vi "DisposeCore.vi"(8 "error in (no error)":errorcluster, 11 "PizzaStore":refnum<class "PizzaStore.lvclass">) -> (0 "error out":errorcluster, 3 "PizzaStore":refnum<class "PizzaStore.lvclass">)   [LabVIEW 2020, in "FactoryMethod.lvlib" / "PizzaFactoryMethod.lvlib" / "PizzaStore.lvclass"]
uses:
  PizzaStore.lvclass
  PizzaStore.lvclass/PizzaStore.ctl
  Private/TypeDef/privateDataDVR.ctl
  Private/TypeDef/privateData.ctl
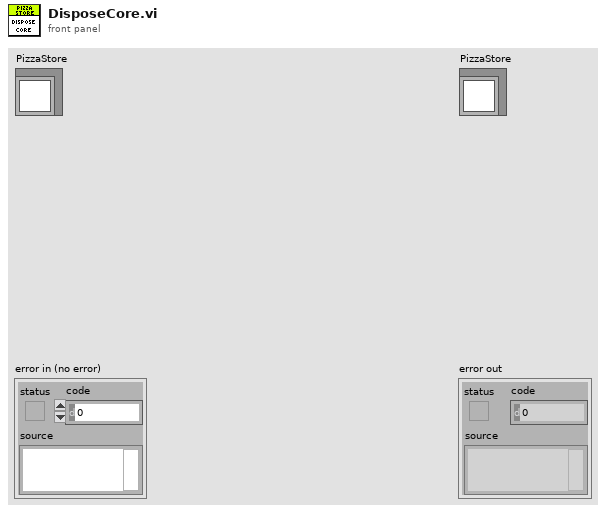
[diagram p1: front panel]
types:
  T1 = typedef "FactoryMethod.lvlib/PizzaFactoryMethod.lvlib/PizzaStore.lvclass/privateDataDVR.ctl" = refnum<data-value>
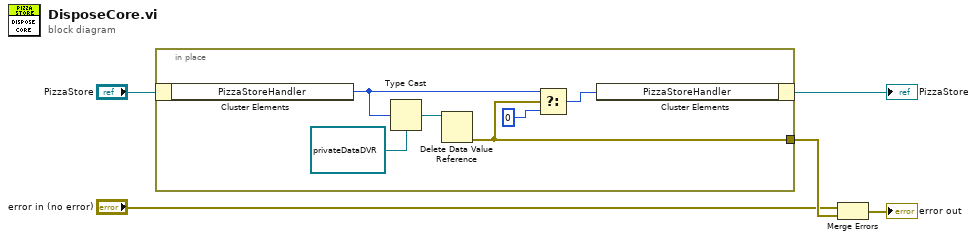
[diagram p0: block diagram]
diagram:
  n1 = in-place {
    in-place-border: [w10] -> w2
    n2 = in-place-cluster #1("PizzaStore") -> ("PizzaStoreHandler"=w9:u32)
    n3 = Type Cast(type=T1 refnum ("privateDataDVR"), x=w9) -> (*(type *) &x=w11:T1)
    n4 = Delete Data Value Reference(data value reference=w11) -> (error out=w10:errorcluster)  [unwired: 1 in, 1 out]
    n5 = Select(t=w9, s=w10, f=u32 0) -> (s? t:f=w8:u32)
    n6 = in-place-cluster #1("PizzaStoreHandler"=w8) -> (→"PizzaStore":refnum<class "PizzaStore.lvclass">)
  }
  n7 = Merge Errors("error in (no error)", w2) -> (→"error out":errorcluster)
